vi "ADC_status_message.vi"(1 "serial poll byte":i16) -> (0 "Status String":string)   [LabVIEW 2010]
panel:
  out "Poll array":bool[](array[boolean])
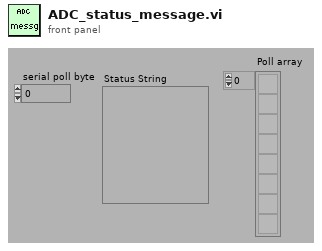
[diagram p1: front panel]
types:
  T1 = cluster{"Boolean array[0]":bool, "Boolean array[1]":bool, "Boolean array[2]":bool, "Boolean array[3]":bool, "Boolean array[4]":bool, "Boolean array[5]":bool, "Boolean array[6]":bool, "Boolean array[7]":bool}
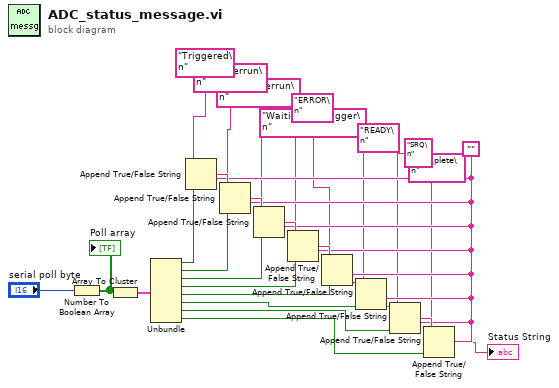
[diagram p0: block diagram]
diagram:
  w13 = ""
  n1 = Number To Boolean Array(number="serial poll byte") -> (Boolean array=w3:bool[])
  "Poll array" <- w3
  n2 = Array To Cluster(array=w3) -> (cluster=w27:T1)
  n3 = Unbundle(w27) -> ("Boolean array[0]"=w20:bool, "Boolean array[1]"=w19:bool, "Boolean array[2]"=w18:bool, "Boolean array[3]"=w17:bool, "Boolean array[4]"=w16:bool, "Boolean array[5]"=w4:bool, "Boolean array[6]"=w15:bool, "Boolean array[7]"=w14:bool)
  n4 = Append True/False String(1:w20, 2:w13, 3:"Triggered\n" ("true string")) -> (0:w26:string)  [unwired: 1 out]
  n5 = Append True/False String(1:w19, 2:w13, 3:"Trig overrun\n" ("true string"), 4:w26) -> (0:w25:string)
  n6 = Append True/False String(1:w18, 2:w13, 3:"Buffer overrun\n" ("true string"), 4:w25) -> (0:w24:string)
  n7 = Append True/False String(1:w17, 2:w13, 3:"ERROR\n" ("true string"), 4:w24) -> (0:w23:string)
  n8 = Append True/False String(1:w16, 2:w13, 3:"Waiting for Trigger\n" ("true string"), 4:w23) -> (0:w22:string)
  n9 = Append True/False String(1:w4, 2:w13, 3:"READY\n" ("true string"), 4:w22) -> (0:w2:string)
  n10 = Append True/False String(1:w15, 2:w13, 3:"SRQ\n" ("true string"), 4:w2) -> (0:w21:string)
  n11 = Append True/False String(1:w14, 2:w13, 3:"Complete\n" ("true string"), 4:w21) -> (0:→"Status String":string)
